vi "lsl child value n.vi"(8 "error in (no error)":errorcluster, 10 "name":string, 11 "e":cluster{}) -> (0 "error out":errorcluster, 2 "function return":string, 3 "e out":cluster{})   [LabVIEW 2016, in "Lab Streaming Layer.lvlib"]
doc: "extern LIBLSL_C_API const char* lsl_child_value_n(lsl_xml_ptr e, const char *name);"
uses:
  Lab Streaming Layer.lvlib
  <userlib>/liblsl-LabVIEW/liblsl64.dll
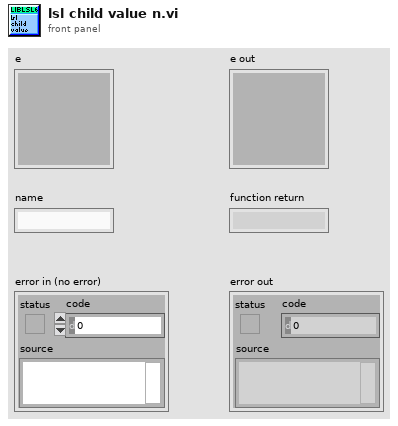
[diagram p1: front panel]
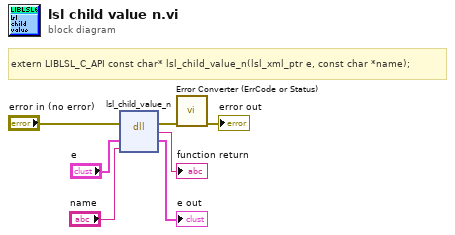
[diagram p0: block diagram]
diagram:
  # "extern LIBLSL_C_API const char* lsl_child_value_n(lsl_xml_ptr e, const char *name);"
  n1 = dll-call lib="C:/Program Files/National Instruments/LabVIEW 2018/user.lib/liblsl-LabVIEW/liblsl64.*" fn="lsl_child_value_n"(error in="error in (no error)", "e"="e", "name"="name") -> (error out=w2:errorcluster, →"function return":string, "e"=→"e out":cluster{})  [unwired: 3 in, 1 out]
  n2 = call "Error Converter (ErrCode or Status).vi"("error in (no error)"=w2) -> ("error out"=→"error out":errorcluster)  [unwired: 10 in]
